vi "test BroadcastRegistry.vi"() -> ()   [LabVIEW 2014]
uses:
  user.lib/_NEVSTOP/JKI State Machine++/_Support/Typedef/_CSM_Broadcast_Response_Message_info.ctl
  user.lib/_NEVSTOP/JKI State Machine++/AdvanceAPI/CSM - Broadcast Message Type.ctl
  user.lib/_NEVSTOP/JKI State Machine++/_Support/FGV-BroadcastRegistry/Operation-BroadcastRegistry.ctl
  user.lib/_NEVSTOP/JKI State Machine++/Communicable State Machine.lvlib
panel:
  out "Response Message Info":T1
  out "Response Message Info":T1
  out "Response Message Info":T1
  out "Response Message Info":T1
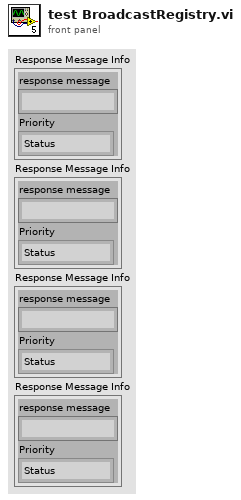
[diagram p1: front panel]
types:
  T1 = typedef "Communicable State Machine.lvlib/_CSM_Broadcast_Response_Message_info.ctl" = cluster{"response message":string, "Priority":T2}
  T2 = typedef "Communicable State Machine.lvlib/CSM - Broadcast Message Type.ctl" = enum16{"Status", "Interrupt(High)"}
  T3 = typedef "Communicable State Machine.lvlib/Operation-BroadcastRegistry.ctl" = enum16{"Delete Source Module", "Delete Target Module", "Remove Module", "Register", "Unregister", "Check"}
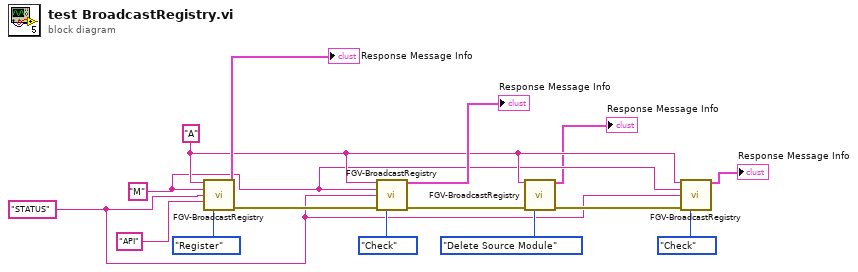
[diagram p0: block diagram]
diagram:
  w3 = "STATUS" ("Message")
  w4 = "M" ("Dest")
  w5 = "A" ("Source")
  n1 = call "FGV-BroadcastRegistry.vi"("Source"=w5, "Target"=w4, "Message"=w3, "Response Message In"="API", "Operation"=Operation-BroadcastRegistry."Register") -> ("Response Message Info"=→"Response Message Info":T1, "Error out"=w12:errorcluster)  [unwired: 8 in, 1 out]
  n2 = call "FGV-BroadcastRegistry.vi"("Source"=w5, "Target"=w4, "Message"=w3, "Error in"=w12, "Operation"=Operation-BroadcastRegistry."Check") -> ("Response Message Info"=→"Response Message Info":T1, "Error out"=w9:errorcluster)  [unwired: 8 in, 1 out]
  n3 = call "FGV-BroadcastRegistry.vi"("Source"=w5, "Error in"=w9, "Operation"=Operation-BroadcastRegistry."Delete Source Module") -> ("Response Message Info"=→"Response Message Info":T1, "Error out"=w6:errorcluster)  [unwired: 10 in, 1 out]
  n4 = call "FGV-BroadcastRegistry.vi"("Source"=w5, "Target"=w4, "Message"=w3, "Error in"=w6, "Operation"=Operation-BroadcastRegistry."Check") -> ("Response Message Info"=→"Response Message Info":T1)  [unwired: 8 in, 2 out]
